vi "TopPortV2.vi"(8 "error in":errorcluster) -> (2 "Shape Report":T1(array[cluster]) {"Score" format="%.2f"; "Centroid"."y" format="%.2f"; "Centroid"."x" format="%.2f"}, 3 "Number of Matches":i32)   [LabVIEW 2019]
uses:
  <vilib>/vision/NI_Vision_Development_Module.lvlib
panel:
  out "x*y":sgl
  out "Mean Value":sgl
  in  "y":sgl
  in  "Minimal Score":dbl=2.0 format="%.2f"
  out "Image Out 2":T2(plugin-control)
  out "Image Out":T2(plugin-control)
  out "error out":errorcluster
  out "Histogram (Histogram 1)":u32[][](array[numeric])
  out "Histogram Graph":u32[][](graph)
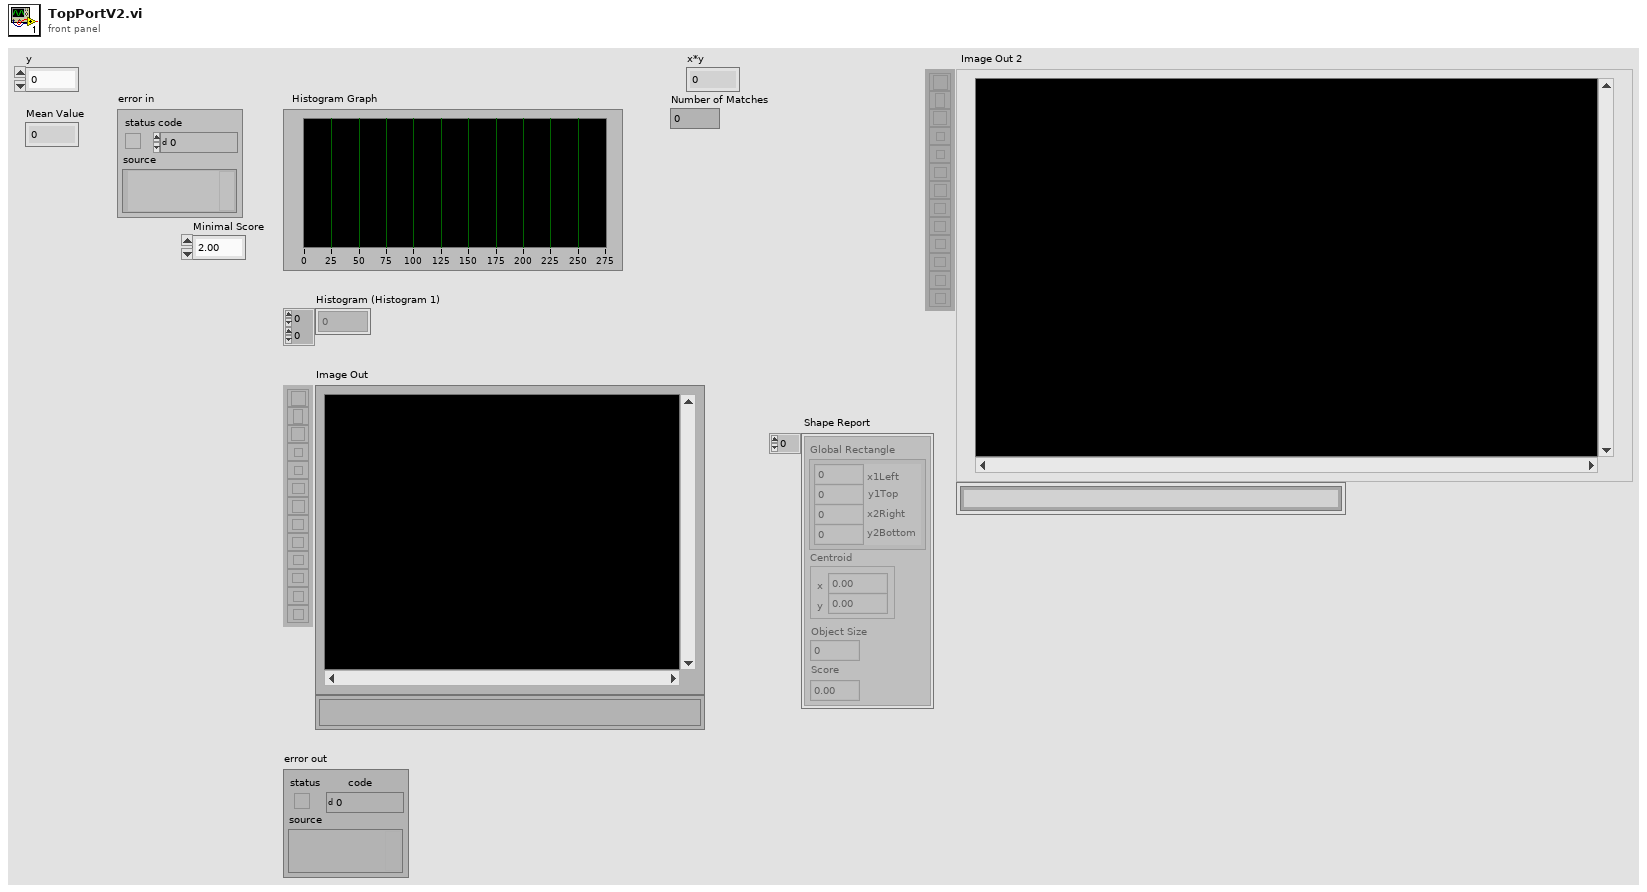
[diagram p1: front panel]
types:
  T1 = cluster{"Global Rectangle":cluster{"x1Left":i32, "y1Top":i32, "x2Right":i32, "y2Bottom":i32}, "Centroid":cluster{"x":sgl, "y":sgl}, "Object Size":u32, "Score":dbl}[]
  T2 = typedef "IMAQ Image.ctl" = refnum<image>
  T3 = cluster{"Measurement Parameter":i32, "Range Lower Value":dbl, "Range Upper Value":dbl, "Range":bool, "Measurement Type":bool}[]
  T4 = enum32{"AutoM", "Close", "Dilate", "Erode", "Gradient", "Gradient in", "Gradient out", "HitMiss", "Open", "PClose", "POpen", "Thick", "Thin"}
  T5 = cluster{"Global Rectangle":i32[], "Contours":cluster{"ID":enum32{"External", "Internal"}, "Type":u32, "Coordinates":i32[]}[]}
  T6 = cluster{"Minimal Value":sgl, "Maximal Value":sgl, "Mean Value":sgl, "Standard  Variation":sgl, "Area (pixels)":i32}
  T7 = cluster{"histogram":u32[], "Minimal Value":sgl, "Maximal Value":sgl, "Starting Value":sgl, "Interval Width":sgl, "Mean Value":sgl, "Standard  Variation":sgl, "Area (pixels)":i32}
  T8 = typedef "Image Type" = u32
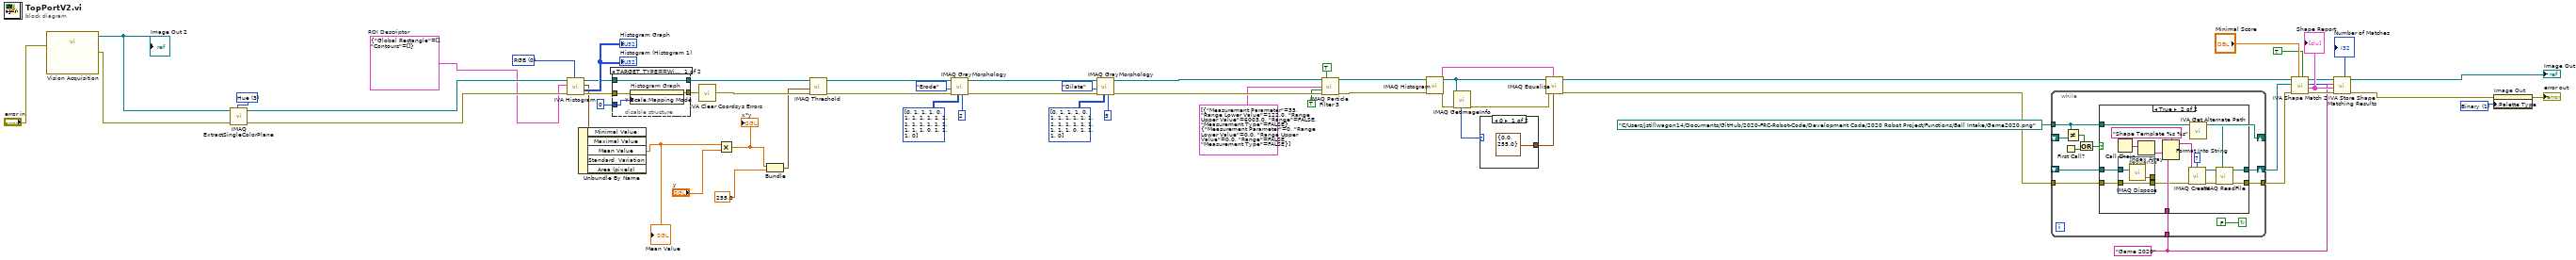
[diagram p0: block diagram]
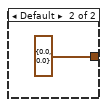
[diagram p3: hidden frame]
diagram:
  w11 = u32 1 items=["Grayscale", "Binary", "Gradient", "Rainbow", "Temperature", "User Defined", "Binary 16 Bit", "Gradient 16 Bit", "Rainbow 16 Bit", "Temperature 16 Bit", "User Defined 16 Bit"] ("Palette Type")
  w14 = "Game 2020" ("Step Name")
  w55 = u16 0 items=["RGB", "HSL", "HSV", "HSI"] ("Color Mode")
  w53 = T5 {"Global Rectangle"=[], "Contours"=[]}  # ROI Descriptor
  w59 = 3 items=["Red", "Green", "Blue", "Hue", "Saturation", "Luminance", "Value", "Intensity"] ("Color Plane")
  n1 = call "Vision Acquisition"("error in"="error in") -> ("Image Out"=w8:T2, "error out"=w10:errorcluster)  [unwired: 25 in]
  "Image Out 2" <- w8
  n2 = call "IMAQ ExtractSingleColorPlane"("Color Plane"=w59, "error in (no error)"=w10, "Image Src"=w8) -> ("error out"=w58:errorcluster, "Image Dst Out"=w57:T2)  [unwired: 1 in, 6 out]
  n3 = call <vilib>:"IVA Histogram.vi"("Color Mode"=w55, "error in (no error)"=w58, "ROI Descriptor"=w53, "Image In"=w57) -> ("error out"=w56:errorcluster, "Histograms"=→"Histogram Graph" →"Histogram (Histogram 1)":u32[][], "Statistics"=w7:T6, "Image Out"=w52:T2)  [unwired: 4 out]
  n4 = Unbundle By Name(w7) -> ("Mean Value"=w5:sgl)  [unwired: 4 out]
  "Mean Value" <- w5
  n5 = disable-structure "Conditional Disable Structure" shown="TARGET_TYPE==Windows" {
    disable-tunnel: w56 -> [w63 w64]
    disable-tunnel: [w62 w64] -> w50
    disable-tunnel: w52 -> [w61 w65]
    disable-tunnel: [w61 w65] -> w48
    disable-tunnel: u8 0 ("Y Scale.Mapping Mode") -> [w60 _]
    frame condition #0 (active) {
      n6 = property on="Histogram Graph" class="WFGraph (strict)"(error in=w63, "Y Scale.Mapping Mode"=w60) -> (error out=w62:errorcluster)  [unwired: 1 in, 1 out]
    }
    frame condition #1 {
    }
  }
  n7 = call <vilib>:"IVA Clear Coordsys Errors.vi"("error in (no error)"=w50) -> ("error out"=w49:errorcluster)  [unwired: 10 in]
  n8 = Multiply(x=w5, y="y") -> (x*y=w3:sgl)
  "x*y" <- w3
  n9 = Bundle(w3, "Upper value"=sgl 255.0) -> (w2:cluster{sgl, "Upper value":sgl})  [unwired: 1 in]
  n10 = call "IMAQ Threshold"("error in (no error)"=w49, "Range"=w2, "Image Src"=w48) -> ("error out"=w47:errorcluster, "Image Dst Out"=w44:T2)  [unwired: 3 in, 4 out]
  n11 = call "IMAQ GrayMorphology"("Number of iterations (1)"=2, "Structuring Element"=i32[][] [[0, 1, 1, 1, 0], [1, 1, 1, 1, 1], [1, 1, 1, 1, 1], [1, 1, 1, 1, 1], [0, 1, 1, 1, 0]], "error in (no error)"=w47, "Operation"=T4."Erode", "Image Src"=w44) -> ("error out"=w43:errorcluster, "Image Dst Out"=w39:T2)  [unwired: 2 in, 3 out]
  n12 = call "IMAQ GrayMorphology"("Number of iterations (1)"=3, "Structuring Element"=i32[][] [[0, 1, 1, 1, 0], [1, 1, 1, 1, 1], [1, 1, 1, 1, 1], [1, 1, 1, 1, 1], [0, 1, 1, 1, 0]], "error in (no error)"=w43, "Operation"=T4."Dilate", "Image Src"=w39) -> ("error out"=w38:errorcluster, "Image Dst Out"=w33:T2)  [unwired: 2 in, 3 out]
  n13 = call "IMAQ Particle Filter 3"("Image Src"=w33, "Connectivity 4/8 (8)"=TRUE, "Selection Values"=T3 [{"Measurement Parameter"=35, "Range Lower Value"=122.0, "Range Upper Value"=6003.0, "Range"=FALSE, "Measurement Type"=FALSE}, {"Measurement Parameter"=0, "Range Lower Value"=0.0, "Range Upper Value"=0.0, "Range"=FALSE, "Measurement Type"=FALSE}], "Keep/Remove Particles (F)"=TRUE ("Keep/Remove Particles"), "error in (no error)"=w38) -> ("Image Dst Out"=w28:T2, "error out"=w34:errorcluster)  [unwired: 4 in, 5 out]
  n14 = call "IMAQ Histogram"("error in (no error)"=w34, "Image"=w28) -> ("error out"=w27:errorcluster, "Histogram Report"=w30:T7)  [unwired: 3 in, 5 out]
  n15 = call "IMAQ GetImageInfo"("error in (no error)"=w27, "Image"=w28) -> ("error out"=w26:errorcluster, "Image Type"=w29:T8)  [unwired: 8 out]
  n16 = case shown="0" w29 {
    tunnel: [cluster{"Minimum":sgl, "Maximum":sgl} {"Minimum"=0.0, "Maximum"=255.0} ("Range") cluster{"Minimum":sgl, "Maximum":sgl} {"Minimum"=0.0, "Maximum"=0.0} ("Range")] -> w25
    frame 0 {
    }
    frame Default {
    }
  }
  n17 = call "IMAQ Equalize"("Range"=w25, "Histogram Report"=w30, "error in (no error)"=w26, "Image Src"=w28) -> ("error out"=w31:errorcluster, "Image Dst Out"=w22:T2)  [unwired: 2 in, 4 out]
  n18 = while {
    shift-right: [w78] -> w15
    shift-left: _ -> [w77]
    tunnel: [w75] -> w16
    tunnel: w31 -> [w74]
    tunnel: path "C:/Users/jstillwagon14/Documents/GitHub/2020-FRC-Robot-Code/Development Code/2020 Robot Project/Functions/Ball Intake/Game2020.png" ("Template Path") -> [w72]
    tunnel: w14 -> [w73]
    shift-right: [w72] -> _
    shift-left: _ -> [w71]
    stop <- FALSE continue-if-true
    n19 = First Call?() -> (First Call?: T/F=w70:bool)
    n20 = Not Equal?(x=w72, y=w71) -> (x != y?=w69:bool)
    n21 = Or(x=w69, y=w70) -> (x .or. y?=w68:bool)
    n22 = case shown="True" w68 {
      tunnel: [w80 w92] -> w78
      tunnel: w77 -> [w80 w83]
      tunnel: [w79 w90] -> w75
      tunnel: w74 -> [w79 w82]
      tunnel: w72 -> [_ w85]
      tunnel: w73 -> [_ w86]
      frame False {
      }
      frame True {
        n23 = Call Chain() -> (call chain=w88:string[])
        n24 = stacked-sequence {
          tunnel: w83 -> [w98]
          tunnel: w82 -> [w97]
          tunnel: [w97] -> w81
          tunnel: [w96] -> _
          frame #0 {
            n25 = call "IMAQ Dispose"("Image"=w98) -> ("error out"=w96:errorcluster)  [unwired: 2 in, 3 out]
          }
        }
        n26 = Index Array(array=w88) -> (element=w87:string)  [unwired: 1 in]
        n27 = Format Into String(format string="Shape Template %s %s" ("Image Name"), w87, w86) -> (resulting string=w95:string)  [unwired: 2 in, 1 out]
        n28 = call "IMAQ Create"("Border Size"=7, "Image Name"=w95, "error in (no error)"=w81) -> ("New Image"=w93:T2, "error out"=w91:errorcluster)  [unwired: 1 in, 1 out]
        n29 = call <vilib>:"IVA Get Alternate Path.vi"("Path In"=w85) -> ("Path Out"=w84:path)  [unwired: 10 out]
        n30 = call "IMAQ ReadFile"("File Path"=w84, "error in (no error)"=w91, "Image"=w93) -> ("error out"=w90:errorcluster, "Image Out"=w92:T2)  [unwired: 2 in, 5 out]
      }
    }
  }
  n31 = call <vilib>:"IVA Shape Match 2.vi"("Scale Invariance"=TRUE, "Minimal Score"="Minimal Score", "error in (no error)"=w16, "Template"=w15, "Image Src"=w22) -> ("error out"=w21:errorcluster, "Shape Report"=w19:T1, "Number of Matches"=→"Number of Matches":i32, "Image Out"=w18:T2)  [unwired: 3 out]
  "Shape Report" <- w19
  n32 = call <vilib>:"IVA Store Shape Matching Results.vi"("error in (no error)"=w21, "Shape Report"=w19, "Step Name"=w14, "Image in"=w18) -> ("error out"=w20:errorcluster, "Image dup"=→"Image Out":T2)  [unwired: 6 out]
  n33 = property on="Image Out" class="ImageControl"(error in=w20, "Palette:Palette Type"=w11) -> (error out=→"error out":errorcluster)  [unwired: 1 in, 1 out]
